vi "Create nipkg Folder Structure.vi"(8 "error in (no error)":errorcluster, 11 "target folder":path) -> (0 "error out":errorcluster, 1 "instructions filepath":path, 2 "control filepath":path, 3 "nipkg unpacked folder":path, 5 "data folderpath":path)   [LabVIEW 2014, in "vipm-to-nipm-package-converter.lvlib"]
doc: "Creates an nipkg folder structure with an empty control file and empty data subfolder. This folder structure can later be packed into a .nipkg file."
uses:
  vipm-to-nipm-package-converter.lvlib
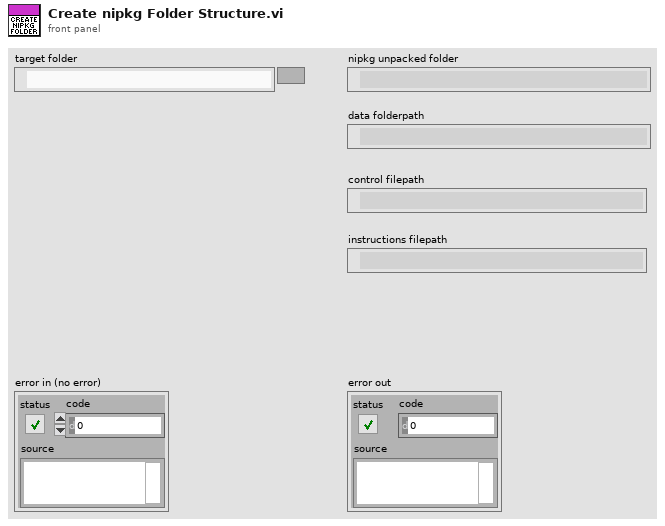
[diagram p1: front panel]
types:
  T1 = enum16{"open", "replace", "create", "open or create", "replace or create", "replace or create with confirmation"}
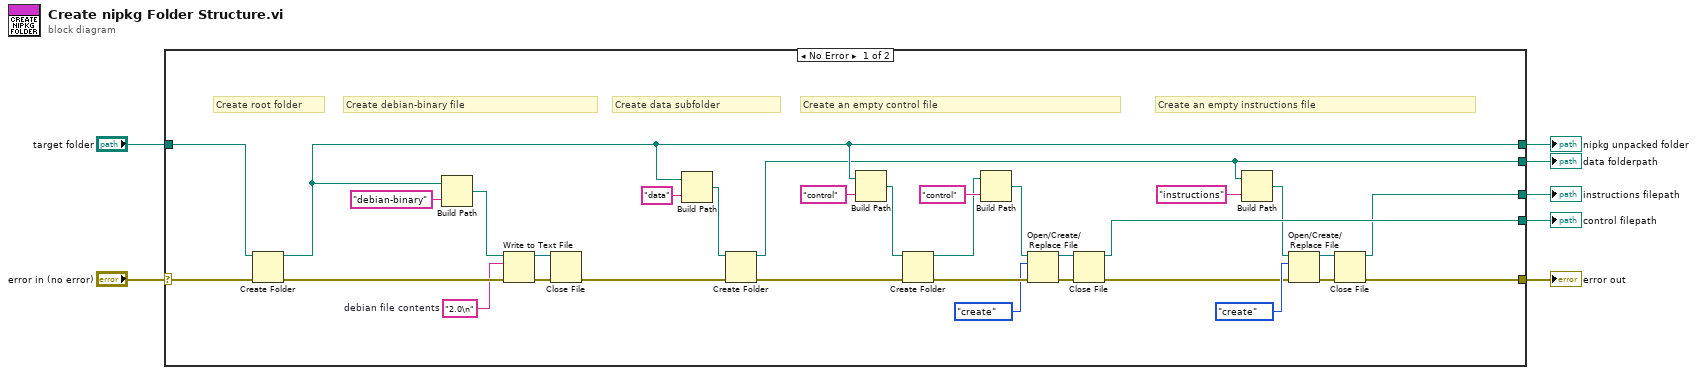
[diagram p0: block diagram]
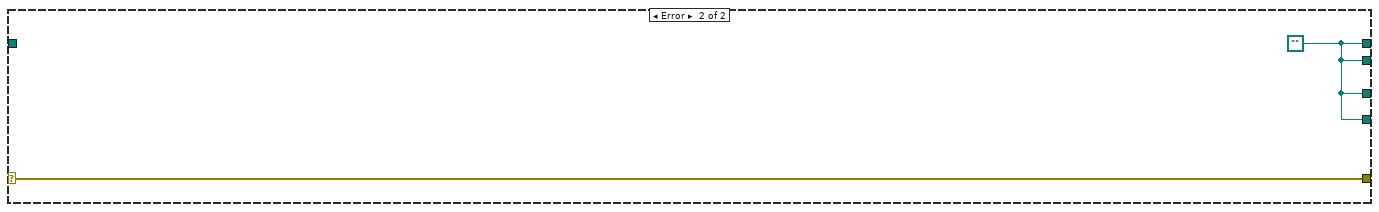
[diagram p2: hidden frame]
diagram:
  n1 = case shown="No Error" "error in (no error)" {
    selector: "error in (no error)" -> [w29 w41]
    tunnel: [w9 w41] -> w7
    tunnel: [w11 w40] -> w6
    tunnel: [w24 w40] -> w5
    tunnel: "target folder" -> [w35 _]
    tunnel: [w17 w40] -> w2
    tunnel: [w8 w40] -> w1
    frame No Error {
      w32 = "2.0\n"  # debian file contents
      # "Create an empty instructions file"
      # "Create an empty control file"
      # "Create data subfolder"
      # "Create debian-binary file"
      # "Create root folder"
      n2 = Create Folder(path (use dialog)=w35, error in=w29) -> (created path=w24:path, error out=w38:errorcluster)  [unwired: 1 in, 1 out]
      n3 = Build Path(base path=w24, name or relative path="debian-binary") -> (appended path=w31:path)
      n4 = Write to Text File(file (use dialog)=w31, text=w32, error in=w38) -> (refnum out=w34:refnum<file>, error out=w33:errorcluster)  [unwired: 1 in, 1 out]
      n5 = Close File(refnum=w34, error in=w33) -> (error out=w39:errorcluster)  [unwired: 1 out]
      n6 = Build Path(base path=w24, name or relative path="data") -> (appended path=w36:path)
      n7 = Create Folder(path (use dialog)=w36, error in=w39) -> (created path=w11:path, error out=w23:errorcluster)  [unwired: 1 in, 1 out]
      n8 = Build Path(base path=w24, name or relative path="control") -> (appended path=w26:path)
      n9 = Create Folder(path (use dialog)=w26, error in=w23) -> (created path=w25:path, error out=w22:errorcluster)  [unwired: 1 in, 1 out]
      n10 = Build Path(base path=w25, name or relative path="control") -> (appended path=w20:path)
      n11 = Open/Create/Replace File(file path (use dialog)=w20, error in=w22, operation (0:open)=T1."create") -> (refnum out=w18:refnum<file>, error out=w21:errorcluster)  [unwired: 3 in, 1 out]
      n12 = Close File(refnum=w18, error in=w21) -> (path=w17:path, error out=w10:errorcluster)
      n13 = Build Path(base path=w11, name or relative path="instructions") -> (appended path=w14:path)
      n14 = Open/Create/Replace File(file path (use dialog)=w14, error in=w10, operation (0:open)=T1."create") -> (refnum out=w16:refnum<file>, error out=w13:errorcluster)  [unwired: 3 in, 1 out]
      n15 = Close File(refnum=w16, error in=w13) -> (path=w8:path, error out=w9:errorcluster)
    }
    frame Error {
      w40 = path ""
    }
  }
  "error out" <- w7
  "data folderpath" <- w6
  "nipkg unpacked folder" <- w5
  "control filepath" <- w2
  "instructions filepath" <- w1
